vi "pulse data FFT.vi"() -> (10 "F output":dbl[][](array[numeric])=[[108.41419421755154, 101.15350847457596], [653.7639068421198, 205.14782370806145], [1300.8217710148638, 50.30141719641081], [1949.7433783291935, 11.890570702296309], [2600.194757386137, 2.642178743768956]] format="%.2f", 15 "peak finder ( F       amp    phase)":string[](array[string]))   [LabVIEW 2016]
uses:
  <vilib>/Analysis/baseanly.llb/Mean (DBL).vi
  <vilib>/Analysis/4window.llb/Hanning Window (DBL).vi
  <vilib>/Analysis/4window.llb/Triangle Window (DBL).vi
  <vilib>/Analysis/4window.llb/Exact Blackman Window (DBL).vi
  <vilib>/Analysis/4window.llb/Flat Top Window (DBL).vi
  <vilib>/Analysis/4window.llb/General Cosine Window (DBL).vi
  <vilib>/Analysis/2dsp.llb/Real FFT.vi
  <vilib>/Analysis/4window.llb/AllCosWindow (DBL).vi
  <vilib>/Analysis/NI_AALPro.lvlib
  <vilib>/Analysis/NI_AALBase.lvlib
panel:
  in  "?":dbl=60.0 format="%.2f"
  in  "Bessel correction?":bool
  in  "save interpolation?":bool
  in  "format":string="%f"
  in  "average traces?":u8=1 min=1 step=1
  in  "save plot?":bool
  in  "format":string="%f"
  in  "threshold / mean":dbl=2.0 format="%.2f"
  out "plotted data":cluster{dbl[], dbl[]}(graph)
  in  "type of interpolation":u16(ring) items=["linear", "cubic spline", "polynomial"]
  in  "no. 1/B interpolation points":u16(ring)=2 items=["1024", "2048", "4096", "8192", "16384", "32768"]
  in  "padding":u16(ring)=2 items=["none", "x 2", "x 4", "x 8"]
  in  "cosine coeffs.":dbl[](array[numeric]) format="%.2f"
  in  "window function":u16(ring)=1 items=["none", "Hanning", "Triangle", "Exact Blackman", "Flat Top", "General Cosine"]
  in  "y domain":u16(ring) items=["channel A"]
  in  "x domain":u16(ring)=3 items=["time (rising field)", "time (falling field)", "1/B (rising field)", "1/B (falling field)", "1/B (rising field + falling field)", "1/B (rising field - falling field)"]
  # "modulation depth (mT)"
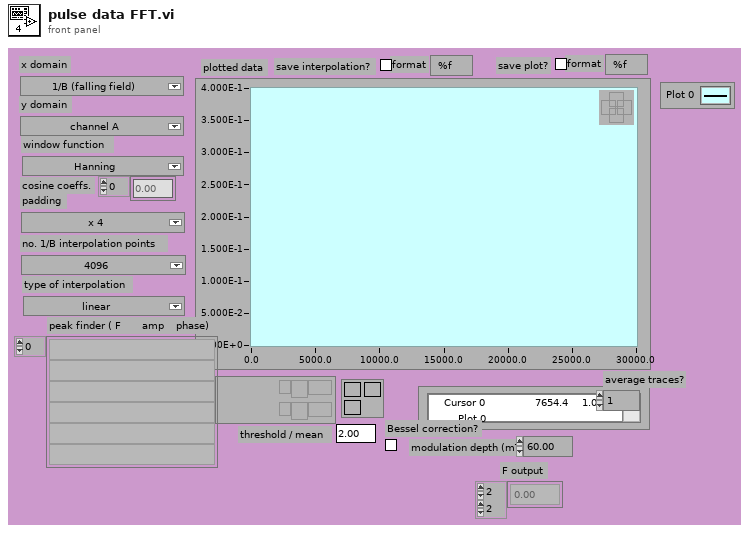
[diagram p1: front panel]
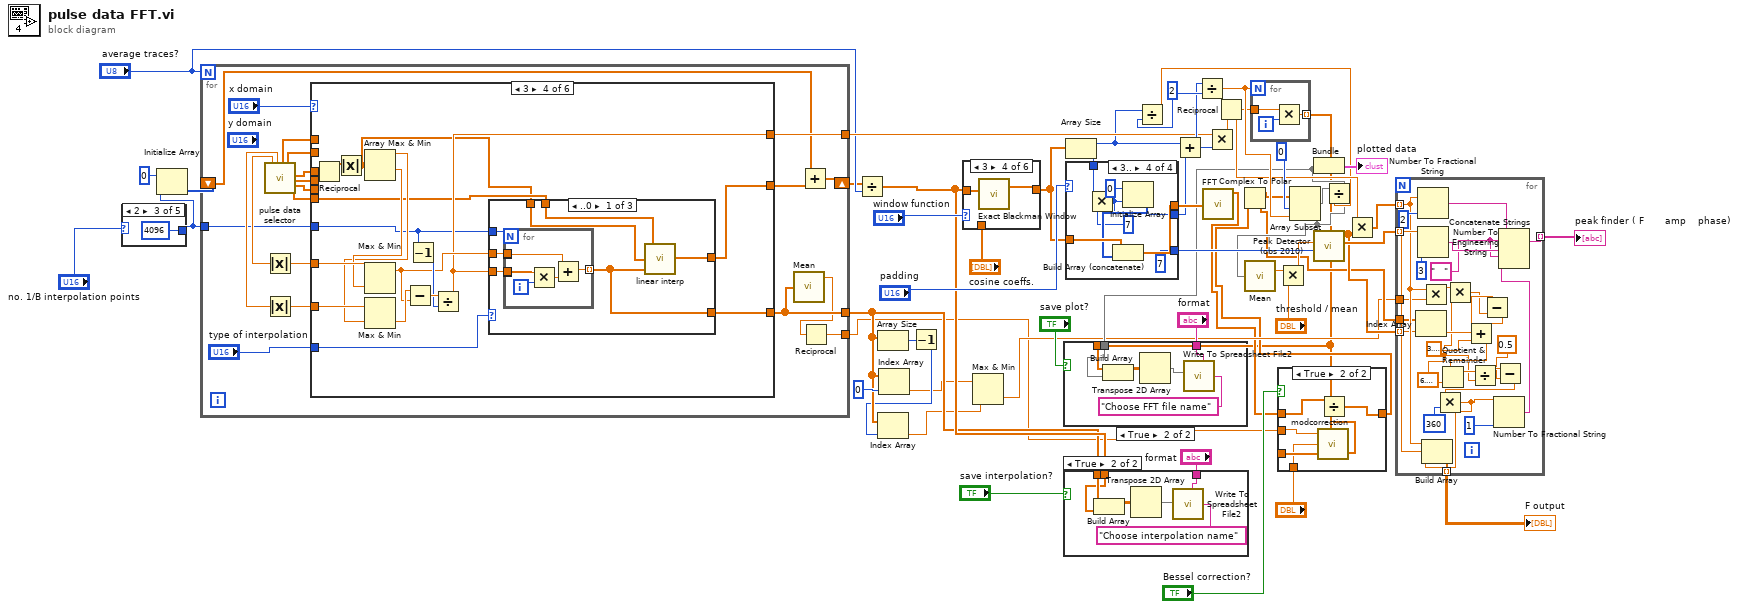
[diagram p0: block diagram]
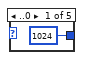
[diagram p4: hidden frame]
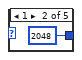
[diagram p5: hidden frame]
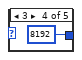
[diagram p6: hidden frame]
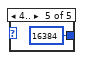
[diagram p7: hidden frame]
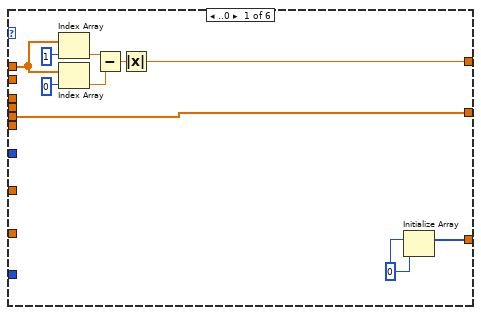
[diagram p8: hidden frame]
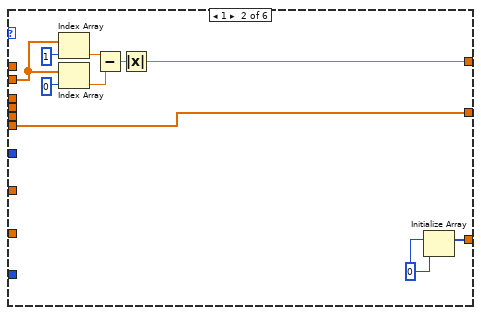
[diagram p9: hidden frame]
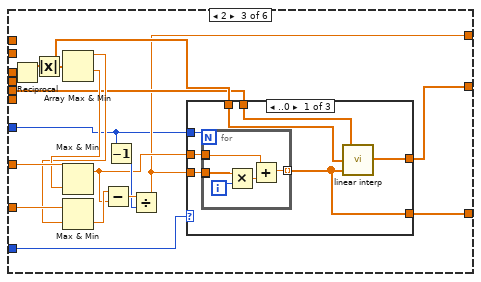
[diagram p10: hidden frame]
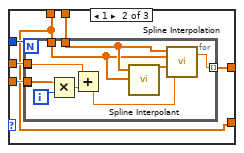
[diagram p11: hidden frame]
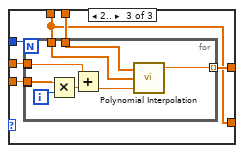
[diagram p12: hidden frame]
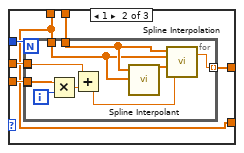
[diagram p13: hidden frame]
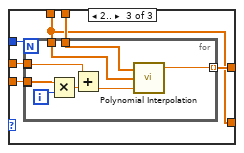
[diagram p14: hidden frame]
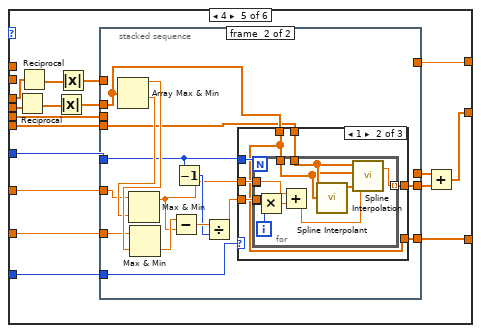
[diagram p15: hidden frame]
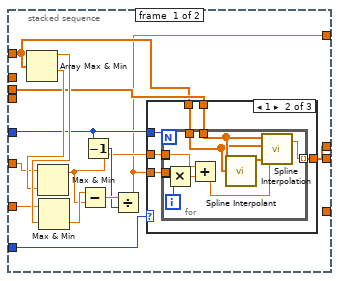
[diagram p16: hidden frame]
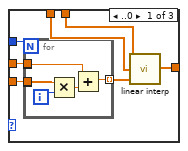
[diagram p17: hidden frame]
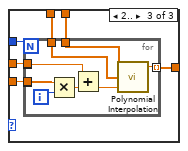
[diagram p18: hidden frame]
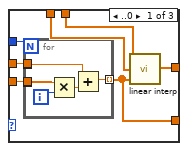
[diagram p19: hidden frame]
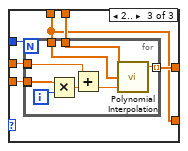
[diagram p20: hidden frame]
diagram:
  w52 = 2
  n1 = case shown="2" "no. 1/B interpolation points" {
    tunnel: [1024 2048 4096 8192 16384] -> w29
    frame ..0 {
    }
    frame 1 {
    }
    frame 2 {
    }
    frame 3 {
    }
    frame 4.. {
    }
  }
  n2 = Initialize Array(0, w29) -> (w28:i32[])
  n3 = for {
    N: "average traces?" -> [_]
    tunnel: w29 -> [w66]
    shift-right: [w62] -> w25
    shift-left: w28 -> [w64]
    tunnel: [w65] -> w27
    tunnel: [w61] -> w11
    tunnel: [w60] -> w3
    n4 = call "pulse data selector.vi"() -> ("1/B start interpolation"=w72:dbl, "1/B end interpolation"=w73:dbl, "time rising"=w68:dbl[], "time falling"=w69:dbl[], "B rising"=w76:dbl[], "B falling"=w77:dbl[], "ch A rising"=w70:dbl[], "ch A falling"=w71:dbl[])  [unwired: 7 in, 5 out]
    n5 = Absolute Value(x=w72) -> (abs(x)=w74:dbl)
    n6 = Absolute Value(x=w73) -> (abs(x)=w75:dbl)
    n7 = case shown="3" "x domain" {
      tunnel: w68 -> [w86 _ _ _ _ _]
      tunnel: w69 -> [_ w92 _ _ _ _]
      tunnel: w70 -> [w82 _ w104 _ w225 w353]
      tunnel: w71 -> [_ w91 _ w161 w226 w354]
      tunnel: [w82 w91 w103 w164 w217 w345] -> w63
      tunnel: [w81 w93 w102 w163 w221 w349] -> w65
      tunnel: w66 -> [_ _ w100 w158 w216 w344]
      tunnel: w74 -> [_ _ w114 w173 w228 w356]
      tunnel: w75 -> [_ _ w112 w171 w227 w355]
      tunnel: w76 -> [_ _ w107 _ w223 w351]
      tunnel: w77 -> [_ _ _ w162 w230 w358]
      tunnel: "type of interpolation" -> [_ _ w106 w166 w229 w357]
      tunnel: [w79 w89 w99 w157 w215 w343] -> w61
      frame ..0 {
        w80 = 0
        n8 = Index Array(array=w86, index=1) -> (element=w85:dbl)
        n9 = Index Array(array=w86, index=0) -> (element=w84:dbl)
        n10 = Subtract(x=w85, y=w84) -> (x-y=w83:dbl)
        n11 = Absolute Value(x=w83) -> (abs(x)=w81:dbl)
        n12 = Initialize Array(w80, w80) -> (w79:i32[])
      }
      frame 1 {
        w90 = 0
        n13 = Index Array(array=w92, index=1) -> (element=w96:dbl)
        n14 = Index Array(array=w92, index=0) -> (element=w95:dbl)
        n15 = Subtract(x=w96, y=w95) -> (x-y=w94:dbl)
        n16 = Absolute Value(x=w94) -> (abs(x)=w93:dbl)
        n17 = Initialize Array(w90, w90) -> (w89:i32[])
      }
      frame 2 {
        n18 = Reciprocal(x=w107) -> (1/x=w101:dbl[])
        n19 = Absolute Value(x=w101) -> (abs(x)=w115:dbl[])
        n20 = Array Max & Min(array=w115) -> (max value=w111:dbl, min value=w113:dbl)  [unwired: 2 out]
        n21 = Max & Min(x=w114, y=w113) -> (max(x,y)=w105:dbl)  [unwired: 1 out]
        n22 = Max & Min(x=w112, y=w111) -> (min(x,y)=w110:dbl)  [unwired: 1 out]
        n23 = Subtract(x=w110, y=w105) -> (x-y=w109:dbl)
        n24 = Decrement(x=w100) -> (x-1=w108:i32)
        n25 = Divide(x=w109, y=w108) -> (x/y=w102:dbl)
        n26 = case shown="..0" w106 {
          tunnel: w100 -> [w122 w133 w148]
          tunnel: w105 -> [w121 w132 w147]
          tunnel: w102 -> [w120 w131 w146]
          tunnel: w115 -> [w118 w128 w143]
          tunnel: w104 -> [w119 w130 w145]
          tunnel: [w117 w129 w144] -> w103
          tunnel: [w116 w128 w143] -> w99
          frame ..0 {
            n27 = for {
              N: w122 -> [_]
              tunnel: [w124] -> _ mode=indexing
              tunnel: [w125] -> _ mode=indexing
              tunnel: w121 -> [w125]
              tunnel: w120 -> [w124]
              tunnel: [w123] -> w116 mode=indexing
              i -> [w127]
              n28 = Multiply(x=w124, y=w127) -> (x*y=w126:dbl)
              n29 = Add(x=w125, y=w126) -> (x+y=w123:dbl)
            }
            n30 = call "linear interp.vi"("x array"=w116, "X data"=w118, "Y data"=w119) -> ("y"=w117:dbl[])
          }
          frame 1 {
            n31 = for {
              N: w133 -> [_]
              tunnel: [w139] -> _ mode=indexing
              tunnel: [w140] -> _ mode=indexing
              tunnel: w132 -> [w140]
              tunnel: w131 -> [w139]
              tunnel: w128 -> [w134]
              tunnel: w130 -> [w138]
              tunnel: [w135] -> w129 mode=indexing
              i -> [w142]
              n32 = Multiply(x=w139, y=w142) -> (x*y=w141:dbl)
              n33 = Add(x=w140, y=w141) -> (x+y=w136:dbl)
              n34 = call <vilib>:"Spline Interpolant.vi"("X"=w134, "Y"=w138) -> ("Interpolant"=w137:dbl[])  [unwired: 2 in, 1 out]
              n35 = call <vilib>:"Spline Interpolation.vi"("x value"=w136, "Interpolant"=w137, "X"=w134, "Y"=w138) -> ("interpolation value"=w135:dbl)  [unwired: 1 out]
            }
          }
          frame 2.. {
            n36 = for {
              N: w148 -> [_]
              tunnel: [w153] -> _ mode=indexing
              tunnel: [w154] -> _ mode=indexing
              tunnel: w147 -> [w154]
              tunnel: w146 -> [w153]
              tunnel: w143 -> [w149]
              tunnel: w145 -> [w152]
              tunnel: [w150] -> w144 mode=indexing
              i -> [w156]
              n37 = Multiply(x=w153, y=w156) -> (x*y=w155:dbl)
              n38 = Add(x=w154, y=w155) -> (x+y=w151:dbl)
              n39 = call <vilib>:"Polynomial Interpolation.vi"("x value"=w151, "X"=w149, "Y"=w152) -> ("interpolation value"=w150:dbl)  [unwired: 2 out]
            }
          }
        }
      }
      frame 3 {
        n40 = Reciprocal(x=w162) -> (1/x=w160:dbl[])
        n41 = Absolute Value(x=w160) -> (abs(x)=w159:dbl[])
        n42 = Array Max & Min(array=w159) -> (max value=w170:dbl, min value=w172:dbl)  [unwired: 2 out]
        n43 = Max & Min(x=w173, y=w172) -> (max(x,y)=w165:dbl)  [unwired: 1 out]
        n44 = Max & Min(x=w171, y=w170) -> (min(x,y)=w169:dbl)  [unwired: 1 out]
        n45 = Subtract(x=w169, y=w165) -> (x-y=w168:dbl)
        n46 = Decrement(x=w158) -> (x-1=w167:i32)
        n47 = Divide(x=w168, y=w167) -> (x/y=w163:dbl)
        n48 = case shown="..0" w166 {
          tunnel: w158 -> [w180 w191 w206]
          tunnel: w165 -> [w179 w190 w205]
          tunnel: w163 -> [w178 w189 w204]
          tunnel: w159 -> [w176 w186 w201]
          tunnel: w161 -> [w177 w188 w203]
          tunnel: [w175 w187 w202] -> w164
          tunnel: [w174 w186 w201] -> w157
          frame ..0 {
            n49 = for {
              N: w180 -> [_]
              tunnel: [w182] -> _ mode=indexing
              tunnel: [w183] -> _ mode=indexing
              tunnel: w179 -> [w183]
              tunnel: w178 -> [w182]
              tunnel: [w181] -> w174 mode=indexing
              i -> [w185]
              n50 = Multiply(x=w182, y=w185) -> (x*y=w184:dbl)
              n51 = Add(x=w183, y=w184) -> (x+y=w181:dbl)
            }
            n52 = call "linear interp.vi"("x array"=w174, "X data"=w176, "Y data"=w177) -> ("y"=w175:dbl[])
          }
          frame 1 {
            n53 = for {
              N: w191 -> [_]
              tunnel: [w197] -> _ mode=indexing
              tunnel: [w198] -> _ mode=indexing
              tunnel: w190 -> [w198]
              tunnel: w189 -> [w197]
              tunnel: w186 -> [w195]
              tunnel: w188 -> [w196]
              tunnel: [w192] -> w187 mode=indexing
              i -> [w200]
              n54 = Multiply(x=w197, y=w200) -> (x*y=w199:dbl)
              n55 = Add(x=w198, y=w199) -> (x+y=w193:dbl)
              n56 = call <vilib>:"Spline Interpolant.vi"("X"=w195, "Y"=w196) -> ("Interpolant"=w194:dbl[])  [unwired: 2 in, 1 out]
              n57 = call <vilib>:"Spline Interpolation.vi"("x value"=w193, "Interpolant"=w194, "X"=w195, "Y"=w196) -> ("interpolation value"=w192:dbl)  [unwired: 1 out]
            }
          }
          frame 2.. {
            n58 = for {
              N: w206 -> [_]
              tunnel: [w211] -> _ mode=indexing
              tunnel: [w212] -> _ mode=indexing
              tunnel: w205 -> [w212]
              tunnel: w204 -> [w211]
              tunnel: w201 -> [w210]
              tunnel: w203 -> [w209]
              tunnel: [w207] -> w202 mode=indexing
              i -> [w214]
              n59 = Multiply(x=w211, y=w214) -> (x*y=w213:dbl)
              n60 = Add(x=w212, y=w213) -> (x+y=w208:dbl)
              n61 = call <vilib>:"Polynomial Interpolation.vi"("x value"=w208, "X"=w210, "Y"=w209) -> ("interpolation value"=w207:dbl)  [unwired: 2 out]
            }
          }
        }
      }
      frame 4 {
        n62 = Reciprocal(x=w230) -> (1/x=w231:dbl[])
        n63 = Reciprocal(x=w223) -> (1/x=w224:dbl[])
        n64 = Absolute Value(x=w231) -> (abs(x)=w220:dbl[])
        n65 = Absolute Value(x=w224) -> (abs(x)=w222:dbl[])
        n66 = stacked-sequence {
          tunnel: w229 -> [w233 w288]
          tunnel: w228 -> [w239 w295]
          tunnel: w227 -> [w238 w294]
          tunnel: w226 -> [_ w289]
          tunnel: w225 -> [w237 _]
          tunnel: w222 -> [w236 _]
          tunnel: w216 -> [w235 w293]
          tunnel: [_ w292] -> w219
          tunnel: [w232 _] -> w221
          tunnel: w220 -> [_ w290]
          tunnel: [w234 _] -> w218
          tunnel: [_ w287] -> w215
          frame #0 {
            n67 = Array Max & Min(array=w236) -> (max value=w241:dbl, min value=w240:dbl)  [unwired: 2 out]
            n68 = Max & Min(x=w239, y=w240) -> (max(x,y)=w242:dbl)  [unwired: 1 out]
            n69 = Max & Min(x=w238, y=w241) -> (min(x,y)=w243:dbl)  [unwired: 1 out]
            n70 = Subtract(x=w243, y=w242) -> (x-y=w245:dbl)
            n71 = Decrement(x=w235) -> (x-1=w244:i32)
            n72 = Divide(x=w245, y=w244) -> (x/y=w232:dbl)
            n73 = case shown="1" w233 {
              tunnel: w235 -> [w252 w263 w278]
              tunnel: w242 -> [w251 w262 w277]
              tunnel: w232 -> [w250 w261 w276]
              tunnel: w236 -> [w248 w260 w275]
              tunnel: w237 -> [w249 w259 w274]
              tunnel: [w246 w258 w273] -> w234
              frame ..0 {
                n74 = for {
                  N: w252 -> [_]
                  tunnel: [w254] -> _ mode=indexing
                  tunnel: [w255] -> _ mode=indexing
                  tunnel: w251 -> [w255]
                  tunnel: w250 -> [w254]
                  tunnel: [w253] -> w247 mode=indexing
                  i -> [w257]
                  n75 = Multiply(x=w254, y=w257) -> (x*y=w256:dbl)
                  n76 = Add(x=w255, y=w256) -> (x+y=w253:dbl)
                }
                n77 = call "linear interp.vi"("x array"=w247, "X data"=w248, "Y data"=w249) -> ("y"=w246:dbl[])
              }
              frame 1 {
                n78 = for {
                  N: w263 -> [_]
                  tunnel: [w269] -> _ mode=indexing
                  tunnel: [w270] -> _ mode=indexing
                  tunnel: w262 -> [w270]
                  tunnel: w261 -> [w269]
                  tunnel: w260 -> [w267]
                  tunnel: w259 -> [w268]
                  tunnel: [w264] -> w258 mode=indexing
                  i -> [w272]
                  n79 = Multiply(x=w269, y=w272) -> (x*y=w271:dbl)
                  n80 = Add(x=w270, y=w271) -> (x+y=w265:dbl)
                  n81 = call <vilib>:"Spline Interpolant.vi"("X"=w267, "Y"=w268) -> ("Interpolant"=w266:dbl[])  [unwired: 2 in, 1 out]
                  n82 = call <vilib>:"Spline Interpolation.vi"("x value"=w265, "Interpolant"=w266, "X"=w267, "Y"=w268) -> ("interpolation value"=w264:dbl)  [unwired: 1 out]
                }
              }
              frame 2.. {
                n83 = for {
                  N: w278 -> [_]
                  tunnel: [w283] -> _ mode=indexing
                  tunnel: [w284] -> _ mode=indexing
                  tunnel: w277 -> [w284]
                  tunnel: w276 -> [w283]
                  tunnel: w275 -> [w282]
                  tunnel: w274 -> [w281]
                  tunnel: [w279] -> w273 mode=indexing
                  i -> [w286]
                  n84 = Multiply(x=w283, y=w286) -> (x*y=w285:dbl)
                  n85 = Add(x=w284, y=w285) -> (x+y=w280:dbl)
                  n86 = call <vilib>:"Polynomial Interpolation.vi"("x value"=w280, "X"=w282, "Y"=w281) -> ("interpolation value"=w279:dbl)  [unwired: 2 out]
                }
              }
            }
          }
          frame #1 {
            n87 = Array Max & Min(array=w290) -> (max value=w297:dbl, min value=w296:dbl)  [unwired: 2 out]
            n88 = Max & Min(x=w295, y=w296) -> (max(x,y)=w298:dbl)  [unwired: 1 out]
            n89 = Max & Min(x=w294, y=w297) -> (min(x,y)=w299:dbl)  [unwired: 1 out]
            n90 = Subtract(x=w299, y=w298) -> (x-y=w301:dbl)
            n91 = Decrement(x=w293) -> (x-1=w300:i32)
            n92 = Divide(x=w301, y=w300) -> (x/y=w291:dbl)
            n93 = case shown="1" w288 {
              tunnel: w293 -> [w308 w319 w334]
              tunnel: w298 -> [w307 w318 w333]
              tunnel: w291 -> [w306 w317 w332]
              tunnel: w290 -> [w304 w314 w329]
              tunnel: w289 -> [w305 w316 w331]
              tunnel: [w303 w315 w330] -> w292
              tunnel: [w302 w314 w329] -> w287
              frame ..0 {
                n94 = for {
                  N: w308 -> [_]
                  tunnel: [w310] -> _ mode=indexing
                  tunnel: [w311] -> _ mode=indexing
                  tunnel: w307 -> [w311]
                  tunnel: w306 -> [w310]
                  tunnel: [w309] -> w302 mode=indexing
                  i -> [w313]
                  n95 = Multiply(x=w310, y=w313) -> (x*y=w312:dbl)
                  n96 = Add(x=w311, y=w312) -> (x+y=w309:dbl)
                }
                n97 = call "linear interp.vi"("x array"=w302, "X data"=w304, "Y data"=w305) -> ("y"=w303:dbl[])
              }
              frame 1 {
                n98 = for {
                  N: w319 -> [_]
                  tunnel: [w325] -> _ mode=indexing
                  tunnel: [w326] -> _ mode=indexing
                  tunnel: w318 -> [w326]
                  tunnel: w317 -> [w325]
                  tunnel: w314 -> [w323]
                  tunnel: w316 -> [w324]
                  tunnel: [w320] -> w315 mode=indexing
                  i -> [w328]
                  n99 = Multiply(x=w325, y=w328) -> (x*y=w327:dbl)
                  n100 = Add(x=w326, y=w327) -> (x+y=w321:dbl)
                  n101 = call <vilib>:"Spline Interpolant.vi"("X"=w323, "Y"=w324) -> ("Interpolant"=w322:dbl[])  [unwired: 2 in, 1 out]
                  n102 = call <vilib>:"Spline Interpolation.vi"("x value"=w321, "Interpolant"=w322, "X"=w323, "Y"=w324) -> ("interpolation value"=w320:dbl)  [unwired: 1 out]
                }
              }
              frame 2.. {
                n103 = for {
                  N: w334 -> [_]
                  tunnel: [w339] -> _ mode=indexing
                  tunnel: [w340] -> _ mode=indexing
                  tunnel: w333 -> [w340]
                  tunnel: w332 -> [w339]
                  tunnel: w329 -> [w338]
                  tunnel: w331 -> [w337]
                  tunnel: [w335] -> w330 mode=indexing
                  i -> [w342]
                  n104 = Multiply(x=w339, y=w342) -> (x*y=w341:dbl)
                  n105 = Add(x=w340, y=w341) -> (x+y=w336:dbl)
                  n106 = call <vilib>:"Polynomial Interpolation.vi"("x value"=w336, "X"=w338, "Y"=w337) -> ("interpolation value"=w335:dbl)  [unwired: 2 out]
                }
              }
            }
          }
        }
        n107 = Add(x=w218, y=w219) -> (x+y=w217:dbl[])
      }
      frame 5.. {
        n108 = Reciprocal(x=w358) -> (1/x=w359:dbl[])
        n109 = Reciprocal(x=w351) -> (1/x=w352:dbl[])
        n110 = Absolute Value(x=w359) -> (abs(x)=w348:dbl[])
        n111 = Absolute Value(x=w352) -> (abs(x)=w350:dbl[])
        n112 = stacked-sequence {
          tunnel: w357 -> [w360 w416]
          tunnel: w356 -> [w367 w423]
          tunnel: w355 -> [w366 w422]
          tunnel: w354 -> [_ w417]
          tunnel: w353 -> [w365 _]
          tunnel: w350 -> [w364 _]
          tunnel: w344 -> [w363 w421]
          tunnel: [_ w420] -> w347
          tunnel: [w361 _] -> w349
          tunnel: w348 -> [_ w418]
          tunnel: [w362 _] -> w346
          tunnel: [_ w415] -> w343
          frame #0 {
            n113 = Array Max & Min(array=w364) -> (max value=w369:dbl, min value=w368:dbl)  [unwired: 2 out]
            n114 = Max & Min(x=w367, y=w368) -> (max(x,y)=w370:dbl)  [unwired: 1 out]
            n115 = Max & Min(x=w366, y=w369) -> (min(x,y)=w371:dbl)  [unwired: 1 out]
            n116 = Subtract(x=w371, y=w370) -> (x-y=w373:dbl)
            n117 = Decrement(x=w363) -> (x-1=w372:i32)
            n118 = Divide(x=w373, y=w372) -> (x/y=w361:dbl)
            n119 = case shown="1" w360 {
              tunnel: w363 -> [w380 w391 w406]
              tunnel: w370 -> [w379 w390 w405]
              tunnel: w361 -> [w378 w389 w404]
              tunnel: w364 -> [w376 w388 w403]
              tunnel: w365 -> [w377 w387 w402]
              tunnel: [w374 w386 w401] -> w362
              frame ..0 {
                n120 = for {
                  N: w380 -> [_]
                  tunnel: [w382] -> _ mode=indexing
                  tunnel: [w383] -> _ mode=indexing
                  tunnel: w379 -> [w383]
                  tunnel: w378 -> [w382]
                  tunnel: [w381] -> w375 mode=indexing
                  i -> [w385]
                  n121 = Multiply(x=w382, y=w385) -> (x*y=w384:dbl)
                  n122 = Add(x=w383, y=w384) -> (x+y=w381:dbl)
                }
                n123 = call "linear interp.vi"("x array"=w375, "X data"=w376, "Y data"=w377) -> ("y"=w374:dbl[])
              }
              frame 1 {
                n124 = for {
                  N: w391 -> [_]
                  tunnel: [w397] -> _ mode=indexing
                  tunnel: [w398] -> _ mode=indexing
                  tunnel: w390 -> [w398]
                  tunnel: w389 -> [w397]
                  tunnel: w388 -> [w395]
                  tunnel: w387 -> [w396]
                  tunnel: [w392] -> w386 mode=indexing
                  i -> [w400]
                  n125 = Multiply(x=w397, y=w400) -> (x*y=w399:dbl)
                  n126 = Add(x=w398, y=w399) -> (x+y=w393:dbl)
                  n127 = call <vilib>:"Spline Interpolant.vi"("X"=w395, "Y"=w396) -> ("Interpolant"=w394:dbl[])  [unwired: 2 in, 1 out]
                  n128 = call <vilib>:"Spline Interpolation.vi"("x value"=w393, "Interpolant"=w394, "X"=w395, "Y"=w396) -> ("interpolation value"=w392:dbl)  [unwired: 1 out]
                }
              }
              frame 2.. {
                n129 = for {
                  N: w406 -> [_]
                  tunnel: [w411] -> _ mode=indexing
                  tunnel: [w412] -> _ mode=indexing
                  tunnel: w405 -> [w412]
                  tunnel: w404 -> [w411]
                  tunnel: w403 -> [w410]
                  tunnel: w402 -> [w409]
                  tunnel: [w407] -> w401 mode=indexing
                  i -> [w414]
                  n130 = Multiply(x=w411, y=w414) -> (x*y=w413:dbl)
                  n131 = Add(x=w412, y=w413) -> (x+y=w408:dbl)
                  n132 = call <vilib>:"Polynomial Interpolation.vi"("x value"=w408, "X"=w410, "Y"=w409) -> ("interpolation value"=w407:dbl)  [unwired: 2 out]
                }
              }
            }
          }
          frame #1 {
            n133 = Array Max & Min(array=w418) -> (max value=w425:dbl, min value=w424:dbl)  [unwired: 2 out]
            n134 = Max & Min(x=w423, y=w424) -> (max(x,y)=w426:dbl)  [unwired: 1 out]
            n135 = Max & Min(x=w422, y=w425) -> (min(x,y)=w427:dbl)  [unwired: 1 out]
            n136 = Subtract(x=w427, y=w426) -> (x-y=w429:dbl)
            n137 = Decrement(x=w421) -> (x-1=w428:i32)
            n138 = Divide(x=w429, y=w428) -> (x/y=w419:dbl)
            n139 = case shown="2.." w416 {
              tunnel: w421 -> [w436 w447 w462]
              tunnel: w426 -> [w435 w446 w461]
              tunnel: w419 -> [w434 w445 w460]
              tunnel: w418 -> [w432 w442 w457]
              tunnel: w417 -> [w433 w444 w459]
              tunnel: [w431 w443 w458] -> w420
              tunnel: [w430 w442 w457] -> w415
              frame ..0 {
                n140 = for {
                  N: w436 -> [_]
                  tunnel: [w438] -> _ mode=indexing
                  tunnel: [w439] -> _ mode=indexing
                  tunnel: w435 -> [w439]
                  tunnel: w434 -> [w438]
                  tunnel: [w437] -> w430 mode=indexing
                  i -> [w441]
                  n141 = Multiply(x=w438, y=w441) -> (x*y=w440:dbl)
                  n142 = Add(x=w439, y=w440) -> (x+y=w437:dbl)
                }
                n143 = call "linear interp.vi"("x array"=w430, "X data"=w432, "Y data"=w433) -> ("y"=w431:dbl[])
              }
              frame 1 {
                n144 = for {
                  N: w447 -> [_]
                  tunnel: [w453] -> _ mode=indexing
                  tunnel: [w454] -> _ mode=indexing
                  tunnel: w446 -> [w454]
                  tunnel: w445 -> [w453]
                  tunnel: w442 -> [w451]
                  tunnel: w444 -> [w452]
                  tunnel: [w448] -> w443 mode=indexing
                  i -> [w456]
                  n145 = Multiply(x=w453, y=w456) -> (x*y=w455:dbl)
                  n146 = Add(x=w454, y=w455) -> (x+y=w449:dbl)
                  n147 = call <vilib>:"Spline Interpolant.vi"("X"=w451, "Y"=w452) -> ("Interpolant"=w450:dbl[])  [unwired: 2 in, 1 out]
                  n148 = call <vilib>:"Spline Interpolation.vi"("x value"=w449, "Interpolant"=w450, "X"=w451, "Y"=w452) -> ("interpolation value"=w448:dbl)  [unwired: 1 out]
                }
              }
              frame 2.. {
                n149 = for {
                  N: w462 -> [_]
                  tunnel: [w467] -> _ mode=indexing
                  tunnel: [w468] -> _ mode=indexing
                  tunnel: w461 -> [w468]
                  tunnel: w460 -> [w467]
                  tunnel: w457 -> [w466]
                  tunnel: w459 -> [w465]
                  tunnel: [w463] -> w458 mode=indexing
                  i -> [w470]
                  n150 = Multiply(x=w467, y=w470) -> (x*y=w469:dbl)
                  n151 = Add(x=w468, y=w469) -> (x+y=w464:dbl)
                  n152 = call <vilib>:"Polynomial Interpolation.vi"("x value"=w464, "X"=w466, "Y"=w465) -> ("interpolation value"=w463:dbl)  [unwired: 2 out]
                }
              }
            }
          }
        }
        n153 = Subtract(x=w346, y=w347) -> (x-y=w345:dbl[])
      }
    }
    n154 = call-poly <vilib>:"Mean.vi"("X"=w61) -> ("mean"=w59:dbl)  [unwired: 1 out]
    n155 = Add(x=w64, y=w63) -> (x+y=w62:dbl[])
    n156 = Reciprocal(x=w59) -> (1/x=w60:dbl)
  }
  n157 = Divide(x=w25, y="average traces?") -> (x/y=w23:dbl[])
  n158 = Array Size(array=w11) -> (size(s)=w12:i32)
  n159 = Index Array(array=w11, index=0) -> (element=w9:dbl)
  n160 = Decrement(x=w12) -> (x-1=w10:i32)
  n161 = Index Array(array=w11, index=w10) -> (element=w8:dbl)
  n162 = case shown="3" "window function" {
    tunnel: w23 -> [w471 w473 w475 w477 w479 w482]
    tunnel: [w471 w472 w474 w476 w478 w481] -> w46
    tunnel: "cosine coeffs." -> [_ _ _ _ _ w480]
    frame ..0 {
    }
    frame 1 {
      n163 = call-poly <vilib>:"Hanning Window.vi"("X"=w473) -> ("Windowed X"=w472:dbl[])  [unwired: 1 out]
    }
    frame 2 {
      n164 = call-poly <vilib>:"Triangle Window.vi"("X"=w475) -> ("Windowed X"=w474:dbl[])  [unwired: 1 out]
    }
    frame 3 {
      n165 = call-poly <vilib>:"Exact Blackman Window.vi"("X"=w477) -> ("Windowed X"=w476:dbl[])  [unwired: 1 out]
    }
    frame 4 {
      n166 = call-poly <vilib>:"Flat Top Window.vi"("X"=w479) -> ("Windowed X"=w478:dbl[])  [unwired: 1 out]
    }
    frame 5.. {
      n167 = call-poly <vilib>:"General Cosine Window.vi"("Cosine Coefficients"=w480, "X"=w482) -> ("Windowed X"=w481:dbl[])  [unwired: 1 out]
    }
  }
  n168 = Max & Min(x=w9, y=w8) -> (min(x,y)=w7:dbl)  [unwired: 1 out]
  n169 = case shown="True" "save interpolation?" {
    tunnel: "format" -> [_ w486]
    tunnel: w11 -> [_ w485]
    tunnel: w23 -> [_ w484]
    frame False {
    }
    frame True {
      n170 = Build Array(w485, w484) -> (w488:dbl[][])
      n171 = Transpose 2D Array(2D array=w488) -> (transposed array=w487:dbl[][])
      n172 = call "Write To Spreadsheet File2.vi"("dialogue"="Choose interpolation name", "format (%.3f)"=w486, "2D data"=w487) -> ()  [unwired: 5 in, 1 out]
    }
  }
  n173 = Array Size(array=w46) -> (size(s)=w20:i32)
  n174 = case shown="3.." "padding" {
    tunnel: w46 -> [w491 w496 w504 w512]
    tunnel: [w491 w494 w502 w510] -> w51
    tunnel: w20 -> [_ w493 w500 w508]
    tunnel: [0 w493 w499 w507] -> w50
    tunnel: [3 3 5 7] -> w40
    frame ..0 {
    }
    frame 1 {
      n175 = Initialize Array(0, w493) -> (w495:i32[])
      n176 = Build Array (concatenate)(w496, w495) -> (w494:dbl[])
    }
    frame 2 {
      n177 = Multiply(x=w500, y=3) -> (x*y=w499:i32)
      n178 = Initialize Array(0, w499) -> (w503:i32[])
      n179 = Build Array (concatenate)(w504, w503) -> (w502:dbl[])
    }
    frame 3.. {
      n180 = Multiply(x=w508, y=7) -> (x*y=w507:i32)
      n181 = Initialize Array(0, w507) -> (w511:i32[])
      n182 = Build Array (concatenate)(w512, w511) -> (w510:dbl[])
    }
  }
  n183 = Divide(x=w20, y=w52) -> (x/y=w19:dbl)
  n184 = Add(x=w20, y=w50) -> (x+y=w41:i32)
  n185 = Divide(x=w41, y=w52) -> (x/y=w45:dbl)
  n186 = call-poly <vilib>:"FFT.vi"("X"=w51) -> ("FFT {X}"=w5:cdb[])  [unwired: 9 in, 1 out]
  n187 = Multiply(x=w27, y=w41) -> (x*y=w53:dbl)
  n188 = Reciprocal(x=w53) -> (1/x=w43:dbl)
  n189 = for {
    N: w45 -> [_]
    tunnel: w43 -> [w515]
    tunnel: [w514] -> w1 mode=indexing
    i -> [w516]
    n190 = Multiply(x=w515, y=w516) -> (x*y=w514:dbl)
  }
  n191 = case shown="True" "Bessel correction?" {
    tunnel: w5 -> [w517 w523]
    tunnel: [w517 w522] -> w4
    tunnel: w3 -> [_ w520]
    tunnel: "?" -> [_ w519]
    tunnel: w1 -> [_ w518]
    frame False {
    }
    frame True {
      n192 = call "modcorrection.vi"("frequency (T)"=w518, "mod depth (mT)"=w519, "field (T)"=w520) -> ("J (n)"=w521:dbl[])  [unwired: 1 out]
      n193 = Divide(x=w523, y=w521) -> (x/y=w522:cdb[])
    }
  }
  n194 = Complex To Polar(r * e^(i*theta)=w4) -> (r=w16:dbl[], theta=w14:dbl[])
  n195 = Array Subset(array=w16, index=0, length=w45) -> (w18:dbl[])
  n196 = Divide(x=w18, y=w19) -> (x/y=w17:dbl[])
  n197 = case shown="True" "save plot?" {
    tunnel: "format" -> [_ w527]
    tunnel: w1 -> [_ w526]
    tunnel: w17 -> [_ w525]
    frame False {
    }
    frame True {
      n198 = Build Array(w526, w525) -> (w529:dbl[][])
      n199 = Transpose 2D Array(2D array=w529) -> (transposed array=w528:dbl[][])
      n200 = call "Write To Spreadsheet File2.vi"("dialogue"="Choose FFT file name", "format (%.3f)"=w527, "2D data"=w528) -> ()  [unwired: 5 in, 1 out]
    }
  }
  n201 = call-poly <vilib>:"Mean.vi"("X"=w17) -> ("mean"=w36:dbl)  [unwired: 1 out]
  n202 = Multiply(x=w36, y="threshold / mean") -> (x*y=w35:dbl)
  n203 = Bundle(w1, w17) -> (→"plotted data":cluster{dbl[], dbl[]})  [unwired: 1 in]
  n204 = call <vilib>:"Peak Detector (obs 2010).vi"("width"=w40, "threshold"=w35, "X"=w17) -> ("Amplitudes"=w38:dbl[], "Locations"=w15:dbl[])  [unwired: 4 in, 3 out]
  n205 = Multiply(x=w43, y=w15) -> (x*y=w39:dbl[])
  n206 = for {
    tunnel: w39 -> [w549] mode=indexing
    tunnel: w38 -> [w551] mode=indexing
    tunnel: [w555] -> w37 mode=indexing
    tunnel: [w550] -> w21 mode=indexing
    tunnel: w7 -> [w548]
    tunnel: w15 -> [w547] mode=indexing
    tunnel: w14 -> [w546]
    w534 = 6.283185307179586
    w540 = "   "
    n207 = Index Array(array=w546, index=w547) -> (element=w545:dbl)
    n208 = Number To Fractional String(number=w549, precision (6)=2) -> (F-format string=w556:string)  [unwired: 2 in]
    n209 = Number To Engineering String(2:3, 4:w551) -> (0:w554:string)  [unwired: 2 in]
    n210 = Multiply(x=w549, y=w548) -> (x*y=w537:dbl)
    n211 = Multiply(x=w537, y=w534) -> (x*y=w536:dbl)
    n212 = Subtract(x=w545, y=w536) -> (x-y=w544:dbl)
    n213 = Add(x=w544, y=3.141592653589793) -> (x+y=w542:dbl)
    n214 = Quotient & Remainder(x=w542, y=w534) -> (x-y*floor(x/y)=w535:dbl)  [unwired: 1 out]
    n215 = Divide(x=w535, y=w534) -> (x/y=w533:dbl)
    n216 = Subtract(x=w533, y=0.5) -> (x-y=w531:dbl)
    n217 = Multiply(x=w531, y=360) -> (x*y=w530:dbl)
    n218 = Build Array(w549, w551, w530) -> (w550:dbl[])
    n219 = Number To Fractional String(number=w530, precision (6)=1) -> (F-format string=w538:string)  [unwired: 2 in]
    n220 = Concatenate Strings(w556, w540, w554, w540, w538) -> (w555:string)
  }
  "peak finder ( F       amp    phase)" <- w37
  "F output" <- w21
